vi "Running Average RT Driver VI.vi"(7 "Operation":T1, 11 "Device Reference in":T2 format="%.0x") -> (0 "Error Code":i32)   [LabVIEW 2012, in "Running Average Custom Device.lvlib"]
uses:
  Running Average Custom Device.lvlib
  <vilib>/NI Veristand/Custom Device API/Custom Device Item Ref.ctl
  <vilib>/NI Veristand/Custom Device API/Model Interface Driver VI Operation.ctl
  <vilib>/NI Veristand/Custom Device API/Block Data Reference.ctl
  <vilib>/NI Veristand/Custom Device API/Data Reference.ctl
  <vilib>/NI Veristand/Custom Device API/Data Access Type.ctl
  <vilib>/NI Veristand/Custom Device API/Get Item Property (U32).vi
  <vilib>/NI Veristand/Custom Device API/Get Item Property (String Array).vi
  <vilib>/NI Veristand/Custom Device API/Global Data Refs.vi
  <vilib>/NI Veristand/Custom Device API/Custom Device API.lvlib
  <vilib>/NI Veristand/Custom Device Tools/Custom Device Utility Library/Custom Device Utility Library.lvlib
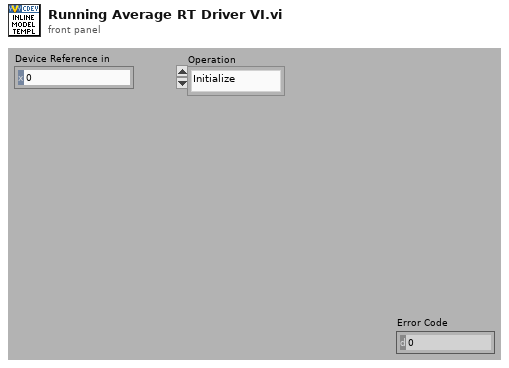
[diagram p1: front panel]
types:
  T1 = typedef "Custom Device API.lvlib/Model Interface Driver VI Operation.ctl" = enum16{"Initialize", "Start", "Execute Model", "Close"}
  T2 = typedef "Custom Device API.lvlib/Custom Device Item Ref.ctl" = u64
  T3 = typedef "Custom Device API.lvlib/Block Data Reference.ctl" = cluster{"Data Reference":T4, "Offset":i32, "Length":i32}
  T4 = typedef "Custom Device API.lvlib/Data Reference.ctl" = i32
  T5 = cluster{"Output Values":dbl[], "Output Block Data Refs":T3[], "Input Values":dbl[], "Input Block Data Refs":T3[], "Channel Buffer":dbl[][], "Index":u32, "Buffer Size":u32, "Reset? Ref":T4, "Buff Elem Used Ref":T4}
  T6 = typedef "Custom Device API.lvlib/Data Access Type.ctl" = enum16{"Read", "Write"}
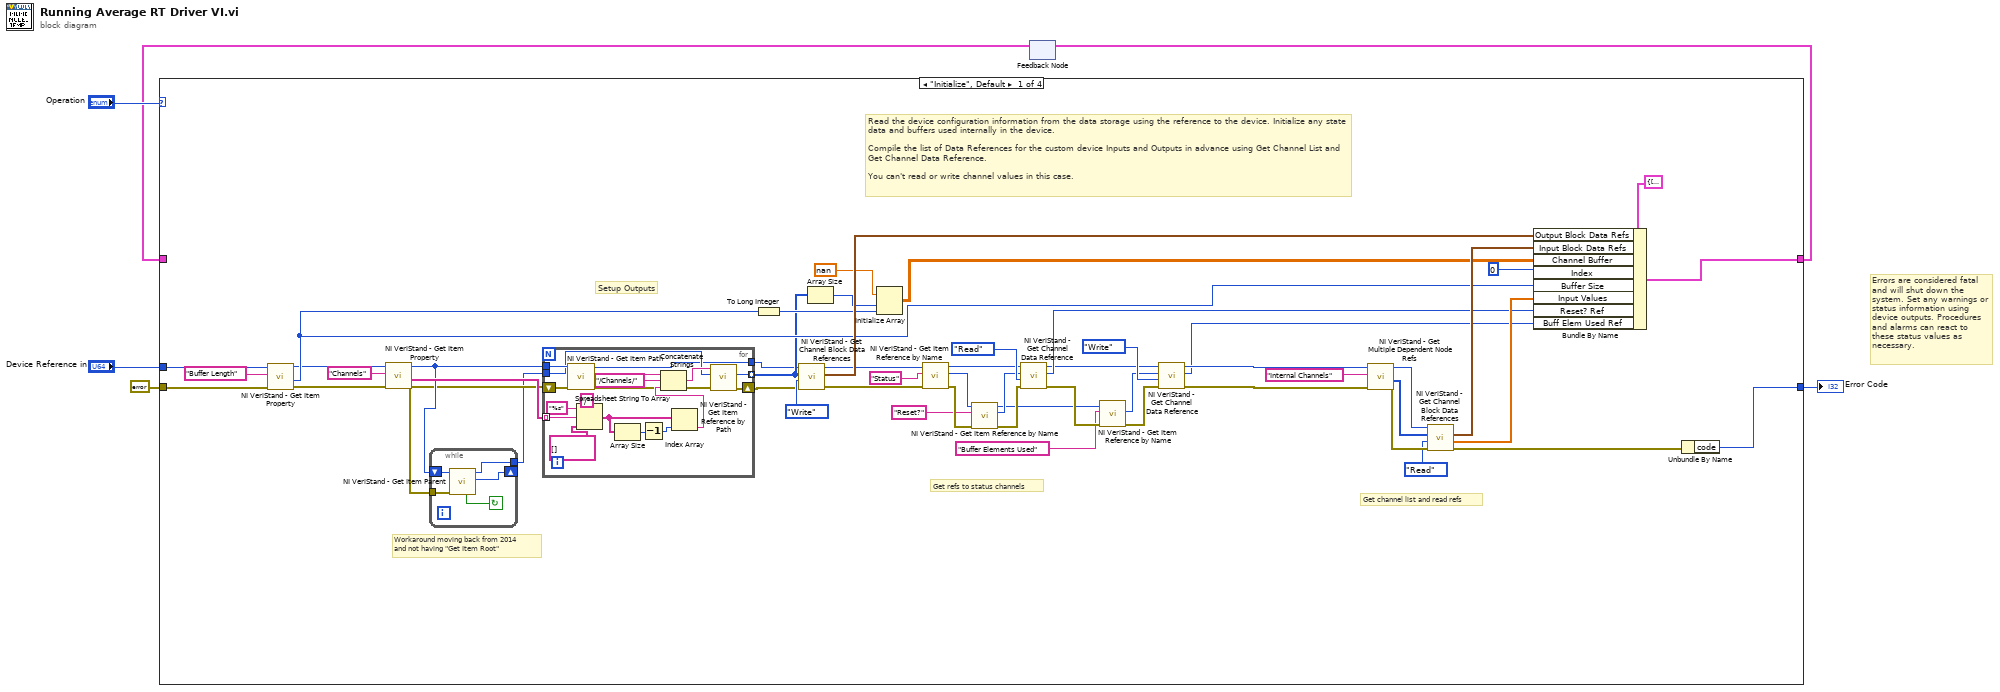
[diagram p0: block diagram]
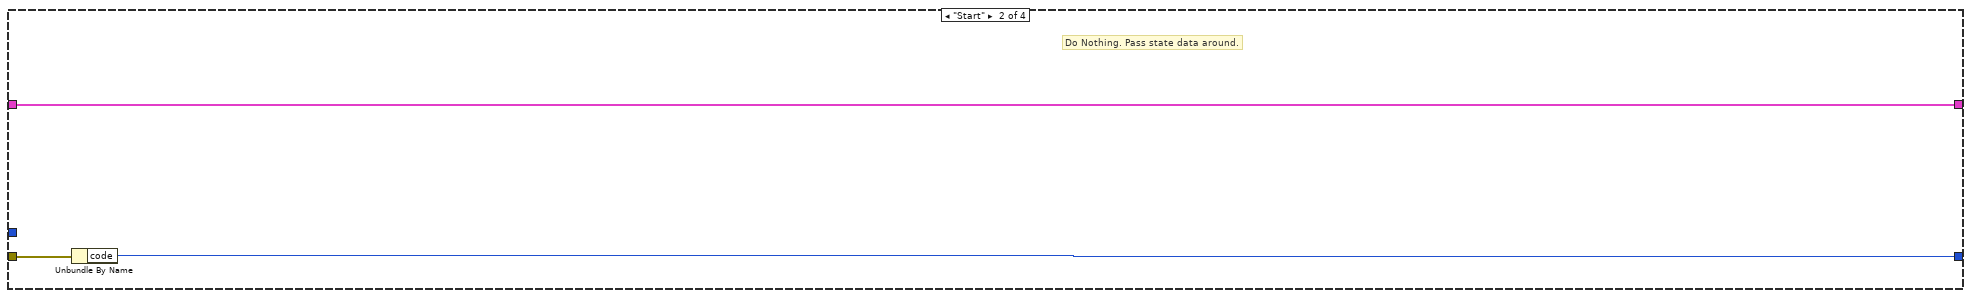
[diagram p2: hidden frame]
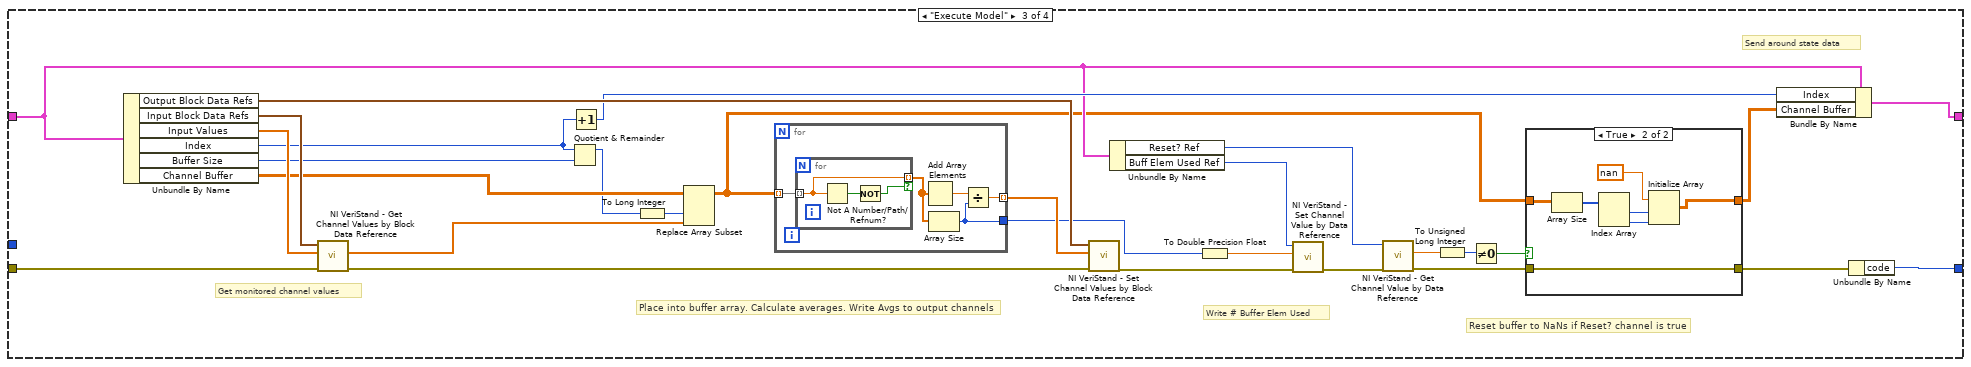
[diagram p3: hidden frame]
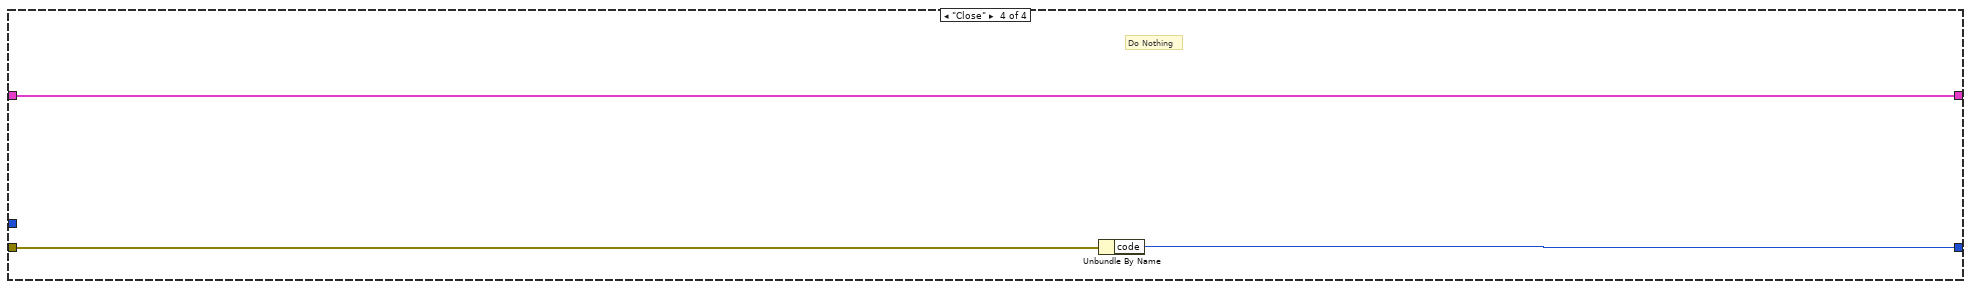
[diagram p5: hidden frame]
diagram:
  # "Errors are considered fatal and will shut down the system. Set any warnings or status information using device outputs. Procedures and alarms can react to these status values as necessary."
  n1 = feedback #1() -> (w4:T5)  [unwired: 1 out]
  n2 = case shown="\"Initialize\", Default" "Operation" {
    tunnel: [w58 w85 w102 w134] -> w5
    tunnel: w4 -> [_ w85 w99 w134]
    tunnel: "Device Reference in" -> [w49 _ _ _]
    tunnel: [w56 w83 w114 w133] -> w3
    tunnel: errorcluster {"status"=FALSE, "code"=0, "source"=""} ("error in (no error)") -> [w48 w84 w111 w132]
    frame "Initialize", Default {
      # "Workaround moving back from 2014\nand not having \"Get Item Root\""
      # "Get refs to status channels"
      # "Get channel list and read refs"
      # "Setup Outputs"
      # "Read the device configuration information from the data storage using the reference to the device. Initialize any state data and buffers used internally in the device.\n\nCompile the list of Data References for the custom device Inputs and Outputs in advance using Get Channel List and Get Channel Data Reference.\n\nYou can't read or write channel values in this case."
      n3 = call-poly <vilib>:"NI VeriStand - Get Item Property.vi"("error in (no error)"=w48, "Property Name"="Buffer Length", "Item Ref in"=w49) -> ("error out"=w36:errorcluster, "Value"=w41:u32, "Item Ref out"=w37:T2)  [unwired: 5 in, 1 out]
      n4 = call-poly <vilib>:"NI VeriStand - Get Item Property.vi"("error in (no error)"=w36, "Property Name"="Channels", "Item Ref in"=w37) -> ("error out"=w8:errorcluster, "Value"=w34:string[], "Item Ref out"=w9:T2)  [unwired: 5 in, 1 out]
      n5 = while {
        shift-right: [w61] -> _
        shift-left: w9 -> [w64]
        tunnel: w8 -> [w63]
        tunnel: [w62] -> w7
        stop <- w60 continue-if-true
        n6 = call <vilib>:"NI VeriStand - Get Item Parent.vi"("error in (no error)"=w63, "Item Ref in"=w64) -> ("Parent Ref"=w61:T2, "Item Ref out"=w62:T2, "Found"=w60:bool)  [unwired: 6 in, 1 out]
      }
      n7 = for {
        tunnel: w9 -> [w82]
        tunnel: w34 -> [w80] mode=indexing
        tunnel: w7 -> [w69]
        tunnel: [w67] -> w33 mode=indexing
        tunnel: [w66] -> w31
        shift-right: [w65] -> w32
        shift-left: w8 -> [w81]
        n8 = call <vilib>:"NI VeriStand - Get Item Path.vi"("error in (no error)"=w81, "Item Ref in"=w82) -> ("error out"=w68:errorcluster, "Path"=w73:string, "Item Ref out"=w66:T2)  [unwired: 6 in, 1 out]
        n9 = Spreadsheet String To Array(delimiter (Tab)="/", format string="%s", spreadsheet string=w80, array type (2D Dbl)=string[] []) -> (array=w75:string[])
        n10 = Array Size(array=w75) -> (size(s)=w76:i32)
        n11 = Decrement(x=w76) -> (x-1=w74:i32)
        n12 = Index Array(array=w75, index=w74) -> (element=w71:string)
        n13 = Concatenate Strings(w73, "/Channels/" ("string"), w71) -> (w70:string)
        n14 = call <vilib>:"NI VeriStand - Get Item Reference by Path.vi"("error in (no error)"=w68, "Root Ref"=w69, "Item Path in"=w70) -> ("error out"=w65:errorcluster, "Item Ref"=w67:T2)  [unwired: 5 in, 2 out]
      }
      n15 = To Long Integer(number=w41) -> (32bit integer=w43:i32)
      n16 = call <vilib>:"NI VeriStand - Get Channel Block Data References.vi"("error in (no error)"=w32, "Access"=Data_Access_Type."Write", "Channel Refs"=w33, "Device Ref in"=w31) -> ("error out"=w25:errorcluster, "Block Data Refs"=w55:T3[], "Device Ref out"=w26:T2)  [unwired: 4 in, 1 out]
      n17 = Array Size(array=w33) -> (size(s)=w45:i32)
      n18 = Initialize Array(nan ("element"), w45, w43) -> (w44:dbl[][])
      n19 = call <vilib>:"NI VeriStand - Get Item Reference by Name.vi"("error in (no error)"=w25, "Item Name"="Status", "Parent Ref in"=w26) -> ("error out"=w20:errorcluster, "Item Ref"=w19:T2, "Parent Ref out"=w21:T2)  [unwired: 5 in, 1 out]
      n20 = call <vilib>:"NI VeriStand - Get Item Reference by Name.vi"("error in (no error)"=w20, "Item Name"="Reset?", "Parent Ref in"=w19) -> ("error out"=w16:errorcluster, "Item Ref"=w17:T2, "Parent Ref out"=w12:T2)  [unwired: 5 in, 1 out]
      n21 = call <vilib>:"NI VeriStand - Get Channel Data Reference.vi"("error in (no error)"=w16, "Access"=Data_Access_Type."Read", "Channel Ref in"=w17, "Device Ref in"=w21) -> ("error out"=w30:errorcluster, "Channel Data Reference"=w24:T4, "Device Ref out"=w10:T2)  [unwired: 5 in]
      n22 = call <vilib>:"NI VeriStand - Get Item Reference by Name.vi"("error in (no error)"=w30, "Item Name"="Buffer Elements Used", "Parent Ref in"=w12) -> ("error out"=w13:errorcluster, "Item Ref"=w11:T2)  [unwired: 5 in, 2 out]
      n23 = call <vilib>:"NI VeriStand - Get Channel Data Reference.vi"("error in (no error)"=w13, "Access"=Data_Access_Type."Write", "Channel Ref in"=w11, "Device Ref in"=w10) -> ("error out"=w28:errorcluster, "Channel Data Reference"=w27:T4, "Device Ref out"=w29:T2)  [unwired: 5 in]
      n24 = call <vilib>:"NI VeriStand - Get Multiple Dependent Node Refs.vi"("error in (no error)"=w28, "Base Property Name"="Internal Channels", "Item Ref in"=w29) -> ("error out"=w54:errorcluster, "Dependent Node Refs"=w53:T2[], "Item Ref out"=w40:T2)  [unwired: 6 in]
      n25 = call <vilib>:"NI VeriStand - Get Channel Block Data References.vi"("error in (no error)"=w54, "Access"=Data_Access_Type."Read", "Channel Refs"=w53, "Device Ref in"=w40) -> ("error out"=w51:errorcluster, "Values Array"=w39:dbl[], "Block Data Refs"=w50:T3[])  [unwired: 4 in, 1 out]
      n26 = Bundle By Name(cluster=T5 {"Output Values"=[], "Output Block Data Refs"=[], "Input Values"=[], "Input Block Data Refs"=[], "Channel Buffer"=[], "Index"=0, "Buffer Size"=0, "Reset? Ref"=0, "Buff Elem Used Ref"=0}, "Output Block Data Refs"=w55, "Input Block Data Refs"=w50, "Channel Buffer"=w44, "Index"=u32 0, "Buffer Size"=w41, "Input Values"=w39, "Reset? Ref"=w24, "Buff Elem Used Ref"=w27) -> (w58:T5)
      n27 = Unbundle By Name(w51) -> ("code"=w56:i32)
    }
    frame "Start" {
      # "Do Nothing. Pass state data around."
      n28 = Unbundle By Name(w84) -> ("code"=w83:i32)
    }
    frame "Execute Model" {
      # "Reset buffer to NaNs if Reset? channel is true"
      # "Write # Buffer Elem Used"
      # "Send around state data"
      # "Place into buffer array. Calculate averages. Write Avgs to output channels"
      # "Get monitored channel values"
      n29 = Unbundle By Name(w99) -> ("Output Block Data Refs"=w106:T3[], "Input Block Data Refs"=w113:T3[], "Input Values"=w112:dbl[], "Index"=w104:u32, "Buffer Size"=w110:u32, "Channel Buffer"=w109:dbl[][])
      n30 = call <vilib>:"NI VeriStand - Get Channel Values by Block Data Reference.vi"("error in (no error)"=w111, "Values Array in"=w112, "Block Data Ref"=w113) -> ("error out"=w105:errorcluster, "Values Array out"=w100:dbl[])  [unwired: 6 in, 1 out]
      n31 = Quotient & Remainder(x=w104, y=w110) -> (x-y*floor(x/y)=w107:u32)  [unwired: 1 out]
      n32 = Increment(x=w104) -> (x+1=w103:u32)
      n33 = To Long Integer(number=w107) -> (32bit integer=w108:i32)
      n34 = Replace Array Subset(array=w109, new element=w100, index (col)=w108) -> (w93:dbl[][])  [unwired: 1 in]
      n35 = for {
        tunnel: w93 -> [w126] mode=indexing
        tunnel: [w127] -> w101 mode=indexing
        tunnel: [w124] -> w89
        n36 = for {
          tunnel: w126 -> [w131] mode=indexing
          tunnel: [w131] -> w125 mode=indexing if=w129
          n37 = Not A Number/Path/Refnum?(number/path/refnum=w131) -> (NaN/Path/Refnum?=w130:bool)
          n38 = Not(x=w130) -> (.not. x?=w129:bool)
        }
        n39 = Add Array Elements(numeric array=w125) -> (sum=w128:dbl)
        n40 = Array Size(array=w125) -> (size(s)=w124:i32)
        n41 = Divide(x=w128, y=w124) -> (x/y=w127:dbl)
      }
      n42 = call <vilib>:"NI VeriStand - Set Channel Values by Block Data Reference.vi"("error in (no error)"=w105, "Values Array in"=w101, "Block Data Ref"=w106) -> ("error out"=w90:errorcluster)  [unwired: 6 in, 2 out]
      n43 = Unbundle By Name(w99) -> ("Reset? Ref"=w98:T4, "Buff Elem Used Ref"=w91:T4)
      n44 = To Double Precision Float(number=w89) -> (double precision float=w88:dbl)
      n45 = call <vilib>:"NI VeriStand - Set Channel Value by Data Reference.vi"("error in (no error)"=w90, "Value"=w88, "Data Reference in"=w91) -> ("error out"=w87:errorcluster)  [unwired: 8 in]
      n46 = call <vilib>:"NI VeriStand - Get Channel Value by Data Reference.vi"("error in (no error)"=w87, "Data Reference in"=w98) -> ("error out"=w94:errorcluster, "Value"=w97:dbl)  [unwired: 8 in]
      n47 = To Unsigned Long Integer(number=w97) -> (unsigned 32bit integer=w96:u32)
      n48 = Not Equal To 0?(x=w96) -> (x != 0?=w95:bool)
      n49 = case shown="True" w95 {
        tunnel: w94 -> [w115 w117]
        tunnel: w93 -> [w116 w123]
        tunnel: [w116 w118] -> w92
        tunnel: [w115 w117] -> w86
        frame False {
        }
        frame True {
          n50 = Array Size(array=w123) -> (size(s)=w122:i32[])
          n51 = Index Array(array=w122) -> (element #1=w120:i32, element #2=w119:i32)  [unwired: 2 in]
          n52 = Initialize Array(nan ("element"), w120, w119) -> (w118:dbl[][])
        }
      }
      n53 = Bundle By Name(cluster=w99, "Index"=w103, "Channel Buffer"=w92) -> (w102:T5)
      n54 = Unbundle By Name(w86) -> ("code"=w114:i32)
    }
    frame "Close" {
      # "Do Nothing"
      n55 = Unbundle By Name(w132) -> ("code"=w133:i32)
    }
  }
  "Error Code" <- w3
  n56 = feedback-in #1(w5) -> ()
